vi "AccNeurons.vi"(2 "No N":i32[](array[numeric])) -> (0 "No N acc":i32[](array[numeric]))   [LabVIEW 2016]
doc: "This VI accumulates the elements in the input array (No neurons). Equal to Matlab funtionn cumsum"
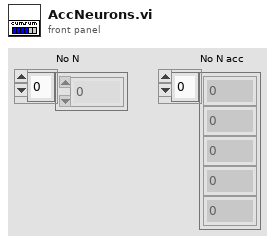
[diagram p1: front panel]
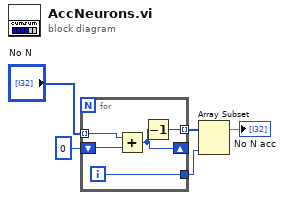
[diagram p0: block diagram]
diagram:
  n1 = for {
    tunnel: "No N" -> [w10] mode=indexing
    shift-right: [w8] -> _
    shift-left: 0 -> [w9]
    tunnel: [w7] -> w3 mode=indexing
    tunnel: [w6] -> w5
    i -> [w6]
    n2 = Add(x=w10, y=w9) -> (x+y=w8:i32)
    n3 = Decrement(x=w8) -> (x-1=w7:i32)
  }
  n4 = Array Subset(array=w3, length=w5) -> (→"No N acc":i32[])  [unwired: 1 in]
